vi "Configuration Reference.vi"(8 "Error in":errorcluster, 11 "Test in":refnum<class "Test.lvclass">) -> (0 "Error out":errorcluster, 1 "Configuration Ref":refnum<vi>, 2 "VI Ref":refnum<vi>, 3 "Test out":refnum<class "Test.lvclass">)   [LabVIEW 2020, in "Test.lvclass"]
doc: "Dynamic method for configuration page reference"
uses:
  Test.lvclass
  Class/INL DNL Test/Test/Children/INL DNL Test/INL DNL Test.lvclass
  Test.lvclass/Test.ctl
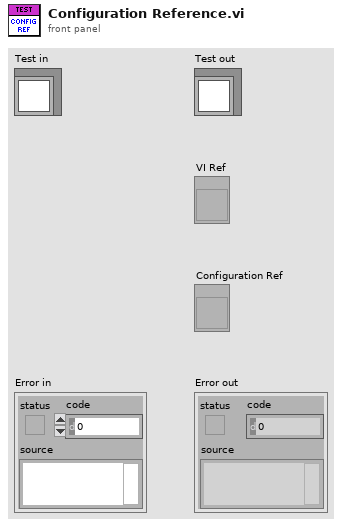
[diagram p1: front panel]
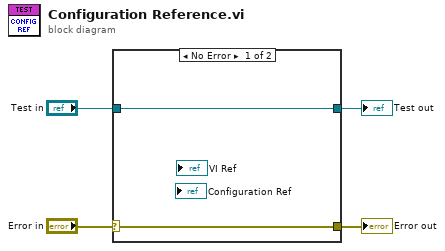
[diagram p0: block diagram]
diagram:
  n1 = case shown="No Error" "Error in" {
    selector: "Error in" -> [w5 w8]
    tunnel: [w5 w8] -> w3
    tunnel: [w6 w7] -> w1
    tunnel: "Test in" -> [w6 w7]
    frame No Error {
    }
    frame Error {
    }
  }
  "Error out" <- w3
  "Test out" <- w1
